vi "ControlAxisSet.vi"(3 "错误输入":errorcluster, 4 "控制电机":T1) -> (0 "错误输出":errorcluster)   [LabVIEW 2018]
panel:
  out "初始化成功成功？":bool
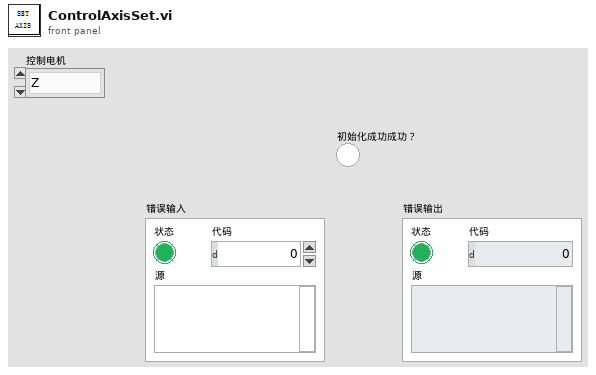
[diagram p1: front panel]
types:
  T1 = typedef "控制电机枚举器.ctl" = enum16{"Z", "Y", "X", "发散角", "俯仰", "旋转"}
  T2 = cluster{"是否停止":enum16{"解除停止", "停止"}, "发生错误停止运行":enum16{"不停止", "停止"}, "发生错误退出运行":enum16{"不退出", "退出"}, "有效电平":cluster{"脉冲信号有效电平":enum16{"低电平有效", "高电平有效"}, "方向信号有效电平 ":enum16{"低电平有效", "高电平有效"}}, "运行脉宽":i32, "加速度和速度边界":cluster{"加速度最大":i32, "速度最大":i32}, "硬件限位设置":cluster{"正限位使能":enum16{"不使能", "使能"}, "正限位极性":enum16{"低电平有效", "高电平有效"}, "负限位使能 ":enum16{"不使能", "使能"}, "负限位极性 ":enum16{"低电平有效", "高电平有效"}}, "伺服报警":cluster{"伺服报警使能":enum16{"不使能", "使能"}, "伺服报警极性":enum16{"低电平有效", "高电平有效"}}, "电机使能":enum16{"不使能", "使能"}, "输出极性":cluster{"寄存器":u32, " fifo":u32, "Bit":u32, "输出极性控制":enum16{"脉冲+方向", "正负脉冲"}}, "运动模式":enum16{"普通模式", "跟踪模式"}, "加速度 puls/s2":i32, "运动速度":cluster{"峰值速度 puls/s":i32, "起始速度puls/s":i32}, "电机速度归一化常量":dbl, "编码器":cluster{"编码器计数模式":enum16{"正交模式", "脉冲+方向模式"}, "编码器计数方向":enum16{"B相超前A相", "A相超前B相"}, "编码器使能":enum16{"不使能", "使能"}, "寄存器位置":i32, "fifo":i32, "data":i32}, "搜零参数":cluster{"orgSW零点开关":enum16{"0开关作为0点", "正限位作为0点", "负限位作为0点"}, "搜零方向":enum16{"正方向", "负方向"}, "零点停止方式":enum16{"立即停止", "减速停止"}, "原点信号边沿":enum16{"下降沿", "上升沿"}, "判断原点位置方向":enum16{"正方向移动", "负方向移动"}, " reducer搜零方式":enum16{"没有减速装置", "原点边缘作为减速", "探针开关作为减速"}, "零点位置":dbl, "搜零高速度":dbl, "搜零低速度":dbl, " 是否等待结束":enum16{"不等待", "等待"}, "编码器索引信号极性":enum16{"下降沿有效", "上升沿有效"}}}
  T3 = cluster{"脉冲信号有效电平":enum16{"低电平有效", "高电平有效"}, "方向信号有效电平 ":enum16{"低电平有效", "高电平有效"}}
  T4 = cluster{"编码器计数模式":enum16{"正交模式", "脉冲+方向模式"}, "编码器计数方向":enum16{"B相超前A相", "A相超前B相"}, "编码器使能":enum16{"不使能", "使能"}, "寄存器位置":i32, "fifo":i32, "data":i32}
  T5 = cluster{"正限位使能":enum16{"不使能", "使能"}, "正限位极性":enum16{"低电平有效", "高电平有效"}, "负限位使能 ":enum16{"不使能", "使能"}, "负限位极性 ":enum16{"低电平有效", "高电平有效"}}
  T6 = cluster{"伺服报警使能":enum16{"不使能", "使能"}, "伺服报警极性":enum16{"低电平有效", "高电平有效"}}
  T7 = cluster{"寄存器":u32, " fifo":u32, "Bit":u32, "输出极性控制":enum16{"脉冲+方向", "正负脉冲"}}
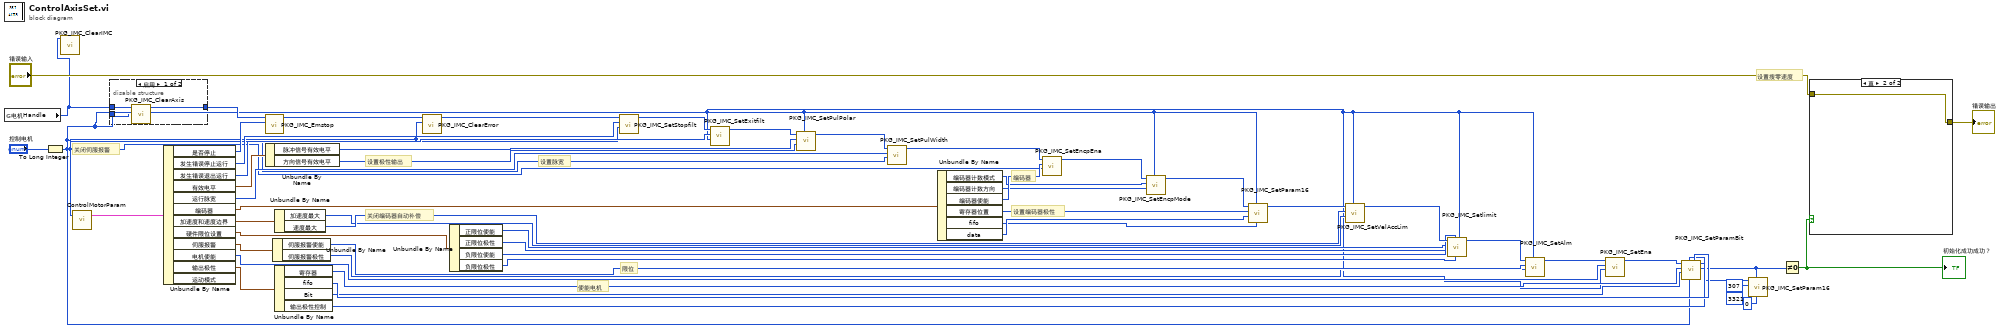
[diagram p0: block diagram]
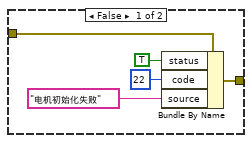
[diagram p3: hidden frame]
diagram:
  # "设置搜零速度"
  # "关闭编码器自动补偿"
  # "设置编码器极性"
  # "设置脉宽"
  # "设置极性输出"
  # "使能电机"
  # "限位"
  # "关闭伺服报警"
  # "编码器"
  n1 = global read "参数.vi" "电机Handle"() -> (w1:u32)
  n2 = To Long Integer(number="控制电机") -> (32bit integer=w7:i32)
  n3 = call "PKG_IMC_ClearIMC.vi"("handle"=w1) -> ()  [unwired: 9 in, 2 out]
  n4 = call "ControlMotorParam.vi"("控制电机"=w7) -> ("轴参数"=w12:T2)  [unwired: 2 in]
  n5 = disable-structure shown="启用" {
    disable-tunnel: w1 -> [w60 w61]
    disable-tunnel: [w59 w61] -> w10
    disable-tunnel: w7 -> [w58 _]
    frame Enabled {
      n6 = call "PKG_IMC_ClearAxis.vi"("axis"=w58, "handle"=w60) -> ("handle out"=w59:u32)  [unwired: 8 in, 1 out]
    }
    frame Disabled {
    }
  }
  n7 = Unbundle By Name(w12) -> ("是否停止"=w8:enum16{"解除停止", "停止"}, "发生错误停止运行"=w57:enum16{"不停止", "停止"}, "发生错误退出运行"=w51:enum16{"不退出", "退出"}, "有效电平"=w50:T3, "运行脉宽"=w48:i32, "编码器"=w24:T4, "加速度和速度边界"=w44:cluster{"加速度最大":i32, "速度最大":i32}, "硬件限位设置"=w41:T5, "伺服报警"=w36:T6, "电机使能"=w33:enum16{"不使能", "使能"}, "输出极性"=w32:T7)  [unwired: 1 out]
  n8 = call "PKG_IMC_Emstop.vi"("isStop"=w8, "Handle"=w10) -> ("Handle out"=w56:u32)  [unwired: 8 in, 1 out]
  n9 = Unbundle By Name(w50) -> ("脉冲信号有效电平"=w13:enum16{"低电平有效", "高电平有效"}, "方向信号有效电平"=w49:enum16{"低电平有效", "高电平有效"})
  n10 = Unbundle By Name(w36) -> ("伺服报警使能"=w35:enum16{"不使能", "使能"}, "伺服报警极性"=w34:enum16{"低电平有效", "高电平有效"})
  n11 = Unbundle By Name(w44) -> ("加速度最大"=w42:i32, "速度最大"=w43:i32)
  n12 = Unbundle By Name(w32) -> ("寄存器"=w31:u32, "fifo"=w30:u32, "Bit"=w28:u32, "输出极性控制"=w29:enum16{"脉冲+方向", "正负脉冲"})
  n13 = call "PKG_IMC_ClearError.vi"("axis"=w7, "Handle"=w56) -> ("Handle out"=w55:u32)  [unwired: 8 in, 1 out]
  n14 = Unbundle By Name(w41) -> ("正限位使能"=w39:enum16{"不使能", "使能"}, "正限位极性"=w38:enum16{"低电平有效", "高电平有效"}, "负限位使能"=w40:enum16{"不使能", "使能"}, "负限位极性"=w37:enum16{"低电平有效", "高电平有效"})
  n15 = call "PKG_IMC_SetStopfilt.vi"("axis"=w7, "stop"=w57, "handle"=w55) -> ("handle out"=w52:u32)  [unwired: 7 in, 1 out]
  n16 = call "PKG_IMC_SetExitfilt.vi"("axis"=w7, "exit"=w51, "handle"=w52) -> ("handle out"=w53:u32)  [unwired: 7 in, 1 out]
  n17 = call "PKG_IMC_SetPulPolar.vi"("axis"=w7, "dir"=w49, "pul"=w13, "handle"=w53) -> ("handle out"=w54:u32)  [unwired: 6 in, 1 out]
  n18 = call "PKG_IMC_SetPulWidth.vi"("axis"=w7, "ns"=w48, "handle"=w54) -> ("handle out"=w22:u32)  [unwired: 7 in, 1 out]
  n19 = Unbundle By Name(w24) -> ("编码器计数模式"=w21:enum16{"正交模式", "脉冲+方向模式"}, "编码器计数方向"=w20:enum16{"B相超前A相", "A相超前B相"}, "编码器使能"=w23:enum16{"不使能", "使能"}, "寄存器位置"=w17:i32, "fifo"=w15:i32, "data"=w16:i32)
  n20 = call "PKG_IMC_SetEncpEna.vi"("axis"=w7, "ena"=w23, "handle"=w22) -> ("handle out"=w19:u32)  [unwired: 7 in, 1 out]
  n21 = call "PKG_IMC_SetEncpMode.vi"("axis"=w7, "dir"=w20, "mode"=w21, "handle"=w19) -> ("handle out"=w18:u32)  [unwired: 6 in, 1 out]
  n22 = call "PKG_IMC_SetParam16.vi"("fifo"=w15, "axis"=w7, "data"=w16, "paramloc"=w17, "Handle"=w18) -> ("Handle out"=w14:u32)  [unwired: 5 in, 1 out]
  n23 = call "PKG_IMC_SetVelAccLim.vi"("axis"=w7, "acclim"=w42, "vellim"=w43, "handle"=w14) -> ("handle out"=w47:u32)  [unwired: 6 in, 1 out]
  n24 = call "PKG_IMC_Setlimit.vi"("axis"=w7, "nlimPolar"=w37, "nlimEna"=w40, "plimPolar"=w38, "plimEna"=w39, "handle"=w47) -> ("handle out"=w46:u32)  [unwired: 4 in, 1 out]
  n25 = call "PKG_IMC_SetAlm.vi"("axis"=w7, "polar"=w34, "ena"=w35, "handle"=w46) -> ("handle out"=w11:u32)  [unwired: 6 in, 1 out]
  n26 = call "PKG_IMC_SetEna.vi"("axis"=w7, "ena"=w33, "handle"=w11) -> ("handle out"=w45:u32)  [unwired: 7 in, 1 out]
  n27 = call "PKG_IMC_SetParamBit.vi"("fifo"=w30, "axis"=w7, "val"=w29, "bit"=w28, "paramloc"=w31, "Handle"=w45) -> ("function return"=w2:i32, "Handle out"=w6:u32)  [unwired: 4 in]
  n28 = call "PKG_IMC_SetParam16.vi"("fifo"=0, "axis"=w2, "data"=i16 3321, "paramloc"=i16 307, "Handle"=w6) -> ()  [unwired: 5 in, 2 out]
  n29 = Not Equal To 0?(x=w2) -> (x != 0?=w27:bool)
  "初始化成功成功？" <- w27
  n30 = case shown="真" w27 {
    tunnel: "错误输入" -> [w66 w67]
    tunnel: [w62 w67] -> w25
    frame False {
      n31 = Bundle By Name(cluster=w66, "status"=TRUE, "code"=22, "source"="电机初始化失败") -> (w62:errorcluster)
    }
    frame True {
    }
  }
  "错误输出" <- w25
